vi "DLTS - run DAQ (SubVI).vi"(5 "Status String Reference":refnum<vi>, 6 "Runs":cluster{"Current run":u32, "Total runs":u32}={"Current run"=1, "Total runs"=1} {"Total runs" min=1; "Current run" min=1}, 7 "Abort Occurrence":refnum<k4>, 8 "error in (no error)":errorcluster, 9 "Timeout 5000ms":u32=5000, 10 "Handle in":T1 {"Handle" format="0x%08x"; "Conn" format="0x%08x"}, 11 "ModHandle in":T2 {"ModHandle" format="0x%08x"; "Conn" format="0x%08x"}) -> (0 "error out":errorcluster, 1 "t":dbl[](array[numeric]), 2 "Samples":dbl[](array[numeric]), 3 "ModHandle Out  out":T2 {"ModHandle" format="0x%08x"; "Conn" format="0x%08x"}, 4 "Aborted":bool)   [LabVIEW 2019]
doc: "Handles DLTS data acquisition"
uses:
  <instrlib>/Zurich Instruments LabOne/Public/Modules/ziTypeModHandle.ctl
  <instrlib>/Zurich Instruments LabOne/Public/ziTypeHandle.ctl
  <instrlib>/Zurich Instruments LabOne/Public/Modules/ziModGetDoubleData.vi
  <instrlib>/Zurich Instruments LabOne/Zurich Instruments LabOne.lvlib
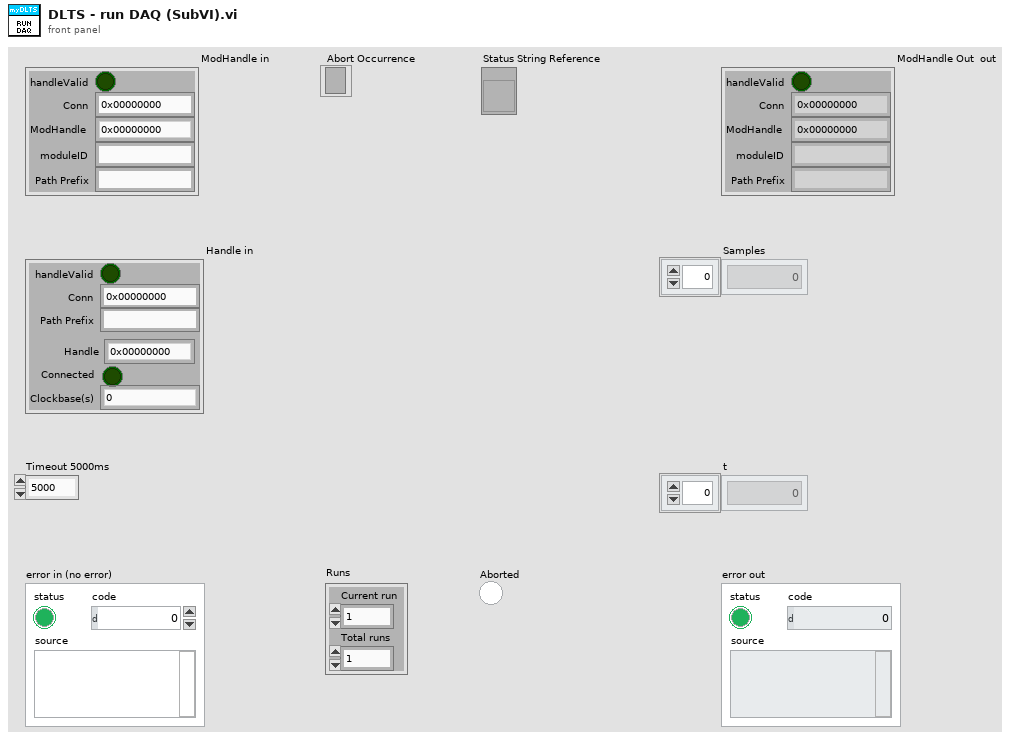
[diagram p1: front panel]
types:
  T1 = typedef "Zurich Instruments LabOne.lvlib/ziTypeHandle.ctl" = cluster{"handleValid":bool, "Conn":u64, "Path Prefix":string, "Handle":u64, "Connected":bool, "Clockbase(s)":dbl}
  T2 = typedef "Zurich Instruments LabOne.lvlib/ziTypeModHandle.ctl" = cluster{"handleValid":bool, "Conn":u64, "ModHandle":u64, "moduleID":string, "Path Prefix":string}
  T3 = typedef "Zurich Instruments LabOne.lvlib/ziTypeModResults.ctl" = cluster{"PathArray":string[], "ValueType":T4, "NoOfResults":u64, "ziGenericHeader":T5[]}
  T4 = typedef "Zurich Instruments LabOne.lvlib/ziTypePollType.ctl" = enum16{"NONE", "DOUBLE_DATA", "INTEGER_DATA", "DEMOD_SAMPLE", "SCOPE_WAVE_HF2", "AUXIN_SAMPLE", "DIO_SAMPLE", "BYTE_ARRAY", "PWA_WAVE", "9", "10", "11", "12", "13", "14", "15", "TREE_CHANGE_DEPRI", "17", "ERROR", "19", "20", "21", "22", "23", "24", "25", "26", "27", "28", "29", "30", "31", "DOUBLE_DATA_TS", "INTEGER_DATA_TS", "34", "SCOPE_WAVE", "SCOPE_WAVE_EX", "37", "BYTE_ARRAY_TS", "39", "40", "41", "42", "43", "44", "45", "CNT_DATA", "47", "TREE_CHANGE", "49", "50", "51", "52", "53", "54", "55", "56", "57", "58", "59", "60", "61", "62", "63", "SWEEPER_DATA", "SPECTRUM_DATA", "ADVISOR_DATA", "VECTOR_DATA", "IMP_DATA", "SHF_GENERATOR_WAVEFORM_DATA", "SHF_RESULT_LOGGER_DATA", "SHF_SCOPE_DATA", "DEMOD_VECTOR"}
  T5 = typedef "Zurich Instruments LabOne.lvlib/ziTypeModGenericHeader.ctl" = cluster{"HeaderType":enum8{"HEADER_TYPE_NONE", "HEADER_TYPE_SWTRIGGER", "HEADER_TYPE_SWEEPER"}, "SampleFormat":u8, "SystemTime":timestamp, "CreatedTimeStamp":u64, "ChangedTimeStamp":u64, "Flags":u32, "ChunkSizeBytes":u64, "Name":string, "Status":u32, "GroupIndex":u32, "Color":u32, "ActiveRow":u32, "TriggerNumber":u64, "GridRows":u32, "GridCols":u32, "GridMode":u32, "GridOperation":u32, "GridDirection":u32, "GridRepetitions":u32, "GridColDelta":dbl, "GridColOffset":dbl, "GridRowDelta":dbl, "GridRowOffset":dbl, "Bandwidth":dbl, "Center":dbl, "Nenbw":dbl}
  T6 = typedef "Zurich Instruments LabOne.lvlib/ziTypeDoubleDataTS.ctl" = cluster{"Timestamp (ticks)":u64[], "Value":dbl[]}
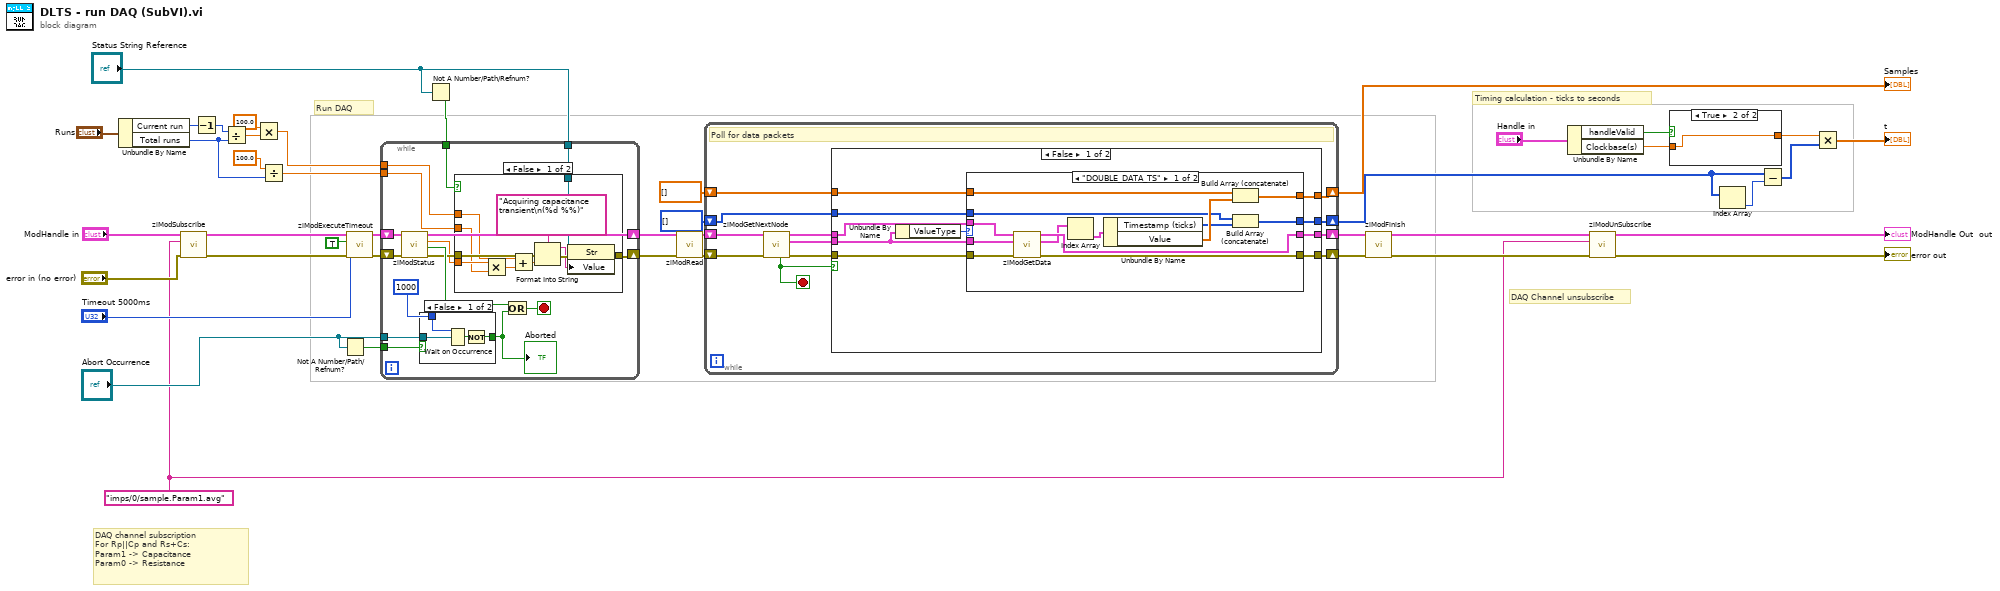
[diagram p0: block diagram]
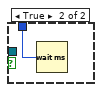
[diagram p2: hidden frame]
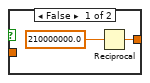
[diagram p6: hidden frame]
diagram:
  w1 = "imps/0/sample.Param1.avg" ("Path")
  # "Timing calculation - ticks to seconds"
  # "DAQ Channel unsubscribe"
  # "DAQ channel subscription\nFor Rp||Cp and Rs+Cs:\nParam1 -> Capacitance\nParam0 -> Resistance"
  # "Run DAQ"
  n1 = Unbundle By Name("Runs") -> ("Current run"=w9:u32, "Total runs"=w4:u32)
  n2 = call <instrlib>:"ziModSubscribe.vi"("Error In"="error in (no error)", "Path"=w1, "ModHandle In"="ModHandle in") -> ("Error Out"=w33:errorcluster, "ModHandle Out"=w32:T2)  [unwired: 6 in]
  n3 = Decrement(x=w9) -> (x-1=w8:u32)
  n4 = Divide(x=w8, y=w4) -> (x/y=w7:dbl)
  n5 = Multiply(x=100.0, y=w7) -> (x*y=w2:dbl)
  n6 = Divide(x=100.0, y=w4) -> (x/y=w3:dbl)
  n7 = Not A Number/Path/Refnum?(number/path/refnum="Abort Occurrence") -> (NaN/Path/Refnum?=w11:bool)
  n8 = call <instrlib>:"ziModExecuteTimeout.vi"("Error In"=w33, "Timeout 5000ms"="Timeout 5000ms", "Modal (F)"=TRUE, "ziModHandle In"=w32) -> ("Error Out"=w20:errorcluster, "ziModHandle Out"=w19:T2)  [unwired: 4 in, 1 out]
  n9 = Not A Number/Path/Refnum?(number/path/refnum="Status String Reference") -> (NaN/Path/Refnum?=w14:bool)
  n10 = while {
    shift-right: [w57] -> w17
    shift-left: w19 -> [w58]
    shift-right: [w49] -> w18
    shift-left: w20 -> [w59]
    tunnel: "Abort Occurrence" -> [w52]
    tunnel: w14 -> [w48]
    tunnel: "Status String Reference" -> [w47]
    tunnel: w11 -> [w46]
    tunnel: w3 -> [w45]
    tunnel: w2 -> [w44]
    stop <- w55 stop-if-true
    n11 = call <instrlib>:"ziModStatus.vi"("Error In"=w59, "ModHandle IN"=w58) -> ("Error Out"=w51:errorcluster, "Finished?"=w56:bool, "Progress (unity)"=w50:dbl, "ModHandle Out"=w57:T2)  [unwired: 5 in]
    n12 = case shown="False" w46 {
      tunnel: [w62 _] -> w54
      tunnel: 1000 ("ms timeout (-1)") -> [w61 w64]
      tunnel: w52 -> [w60 _]
      frame False {
        n13 = Wait on Occurrence(2:w60, 3:w61) -> (0:w63:bool)  [unwired: 1 in]
        n14 = Not(x=w63) -> (.not. x?=w62:bool)
      }
      frame True {
        n15 = Wait (ms)(milliseconds to wait=w64) -> ()  [unwired: 1 out]
      }
    }
    "Aborted" <- w54
    n16 = case shown="False" w48 {
      tunnel: w51 -> [w75 w76]
      tunnel: w50 -> [w73 _]
      tunnel: [w71 w76] -> w49
      tunnel: w47 -> [w69 _]
      tunnel: w45 -> [w68 _]
      tunnel: w44 -> [w65 _]
      frame False {
        n17 = Multiply(x=w73, y=w68) -> (x*y=w66:dbl)
        n18 = Add(x=w65, y=w66) -> (x+y=w67:dbl)
        n19 = Format Into String(format string="Acquiring capacitance transient\n(%d %%)", error in=w75, w67) -> (resulting string=w70:string, error out=w72:errorcluster)  [unwired: 1 in]
        n20 = property class="Str"(reference=w69, error in=w72, "Value"=w70) -> (error out=w71:errorcluster)  [unwired: 1 out]
      }
      frame True {
      }
    }
    n21 = Or(x=w56, y=w54) -> (x .or. y?=w55:bool)
  }
  n22 = call <instrlib>:"ziModRead.vi"("error in"=w18, "ziModHandle In"=w17) -> ("error out"=w15:errorcluster, "ziModHandle Out"=w16:T2)  [unwired: 8 in]
  n23 = while {
    shift-right: [w77] -> w39
    shift-left: w16 -> [w87]
    shift-right: [w82] -> w38
    shift-left: w15 -> [w88]
    shift-right: [w81] -> w37
    shift-left: dbl[] [] -> [w78]
    shift-right: [w79] -> w35
    shift-left: u64[] [] -> [w80]
    stop <- w85 stop-if-true
    # "Poll for data packets"
    n24 = call <instrlib>:"ziModGetNextNode.vi"("Error In"=w88, "ModHandle In"=w87) -> ("Error Out"=w84:errorcluster, "ModResults"=w86:T3, "ModHandle Out"=w83:T2, "NoData"=w85:bool)  [unwired: 6 in]
    n25 = case shown="False" w85 {
      tunnel: w86 -> [w92 _]
      tunnel: w84 -> [w97 w118]
      tunnel: w83 -> [w96 w119]
      tunnel: [w95 w118] -> w82
      tunnel: [w94 w117] -> w81
      tunnel: w78 -> [w93 w117]
      tunnel: [w91 w116] -> w79
      tunnel: w80 -> [w90 w116]
      tunnel: [w89 w119] -> w77
      frame False {
        n26 = Unbundle By Name(w92) -> ("ValueType"=w98:T4)
        n27 = case shown="\"DOUBLE_DATA_TS\"" w98 {
          tunnel: w97 -> [w110 w114]
          tunnel: w96 -> [w111 w115]
          tunnel: [w109 w115] -> w89
          tunnel: [w108 w114] -> w95
          tunnel: [w104 w113] -> w94
          tunnel: w93 -> [w103 w113]
          tunnel: w92 -> [w102 _]
          tunnel: [w100 w112] -> w91
          tunnel: w90 -> [w99 w112]
          frame "DOUBLE_DATA_TS" {
            n28 = call-poly <instrlib>:"ziModGetData.vi"("Error In"=w110, "ModResults"=w102, "ModHandle In"=w111) -> ("Error Out"=w108:errorcluster, "DoubleSample"=w107:T6[], "ModHandle Out"=w109:T2)  [unwired: 4 in, 2 out]
            n29 = Index Array(array=w107) -> (element=w106:T6)  [unwired: 1 in]
            n30 = Unbundle By Name(w106) -> ("Timestamp (ticks)"=w101:u64[], "Value"=w105:dbl[])
            n31 = Build Array (concatenate)(w103, w105) -> (w104:dbl[])
            n32 = Build Array (concatenate)(w99, w101) -> (w100:u64[])
          }
          frame Default {
          }
        }
      }
      frame True {
      }
    }
  }
  "Samples" <- w37
  n33 = call <instrlib>:"ziModFinish.vi"("Error In"=w38, "ziModHandle In"=w39) -> ("Error Out"=w29:errorcluster, "ziModHandle Out"=w40:T2)  [unwired: 7 in]
  n34 = Unbundle By Name("Handle in") -> ("handleValid"=w22:bool, "Clockbase(s)"=w24:dbl)
  n35 = call <instrlib>:"ziModUnSubscribe.vi"("Error In"=w29, "Path (\"/\")"=w1, "ModHandle In"=w40) -> ("Error Out"=→"error out":errorcluster, "ModHandle Out"=→"ModHandle Out  out":T2)  [unwired: 7 in]
  n36 = case shown="True" w22 {
    tunnel: w24 -> [_ w122]
    tunnel: [w121 w122] -> w42
    frame False {
      n37 = Reciprocal(x=210000000.0) -> (1/x=w121:dbl)
    }
    frame True {
    }
  }
  n38 = Index Array(array=w35) -> (element=w36:u64)  [unwired: 1 in]
  n39 = Subtract(x=w35, y=w36) -> (x-y=w41:u64[])
  n40 = Multiply(x=w42, y=w41) -> (x*y=→"t":dbl[])
